vi "Last Conf Save.vi"(7 "error in":errorcluster, 10 "Conf File":path) -> (0 "error out":errorcluster)   [LabVIEW 2019, in "Generic Test Stand.lvclass"]
uses:
  Generic Test Stand.lvclass
  <vilib>/Utility/config.llb/Write Key (String).vi
  <vilib>/Utility/config.llb/NI_LVConfig.lvlib
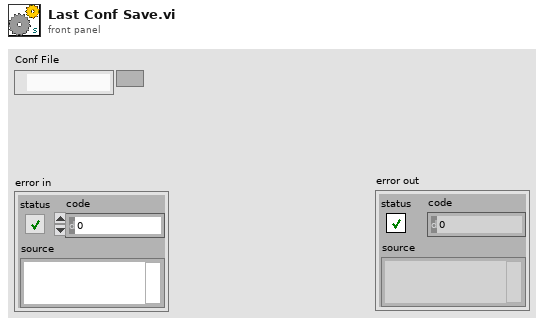
[diagram p1: front panel]
types:
  T1 = typedef "NI_LVConfig.lvlib/Config Data RefNum.ctl" = refnum<k1>
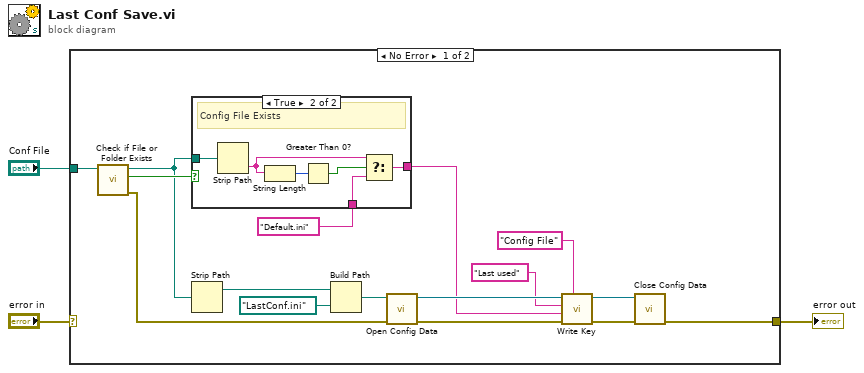
[diagram p0: block diagram]
diagram:
  n1 = case shown="No Error" "error in" {
    selector: "error in" -> [_ w27]
    tunnel: [w11 w27] -> w3
    tunnel: "Conf File" -> [w7 _]
    frame No Error {
      n2 = call <vilib>:"Check if File or Folder Exists.vi"("path"=w7) -> ("error out"=w4:errorcluster, "file or folder exists?"=w8:bool, "dup path"=w6:path)  [unwired: 8 in]
      n3 = case shown="True" w8 {
        tunnel: w6 -> [_ w26]
        tunnel: [w20 w25] -> w9
        tunnel: "Default.ini" -> [w20 w21]
        frame False {
          # "No Config File"
        }
        frame True {
          # "Config File Exists"
          n4 = Strip Path(path=w26) -> (name=w23:string)  [unwired: 1 out]
          n5 = String Length(string=w23) -> (length=w24:i32)
          n6 = Greater Than 0?(x=w24) -> (x > 0?=w22:bool)
          n7 = Select(t=w23, s=w22, f=w21) -> (s? t:f=w25:string)
        }
      }
      n8 = Strip Path(path=w6) -> (stripped path=w5:path)  [unwired: 1 out]
      n9 = Build Path(base path=w5, name or relative path=path "LastConf.ini") -> (appended path=w19:path)
      n10 = call <vilib>:"Open Config Data.vi"("error in (no error)"=w4, "configuration file path"=w19) -> ("error out"=w18:errorcluster, "refnum"=w17:T1)  [unwired: 7 in, 1 out]
      n11 = call-poly <vilib>:"Write Key.vi"("section"="Config File", "error in (no error)"=w18, "value"=w9, "key"="Last used", "refnum"=w17) -> ("error out"=w12:errorcluster, "refnum out"=w13:T1)  [unwired: 4 in, 1 out]
      n12 = call <vilib>:"Close Config Data.vi"("error in (no error)"=w12, "refnum"=w13) -> ("error out"=w11:errorcluster)  [unwired: 8 in, 1 out]
    }
    frame Error {
    }
  }
  "error out" <- w3
